vi "Write tSensorOnTreeElements_Core.vi"(8 "error in (no error)":errorcluster, 9 "System_settings IN":T1={"Units in the system"=[], "dBase names by units"=[], "TCP/IP processing units addresses"=[], "TCP/IP server address"="", "dBase User Name_Cli"="codis_cli", "dBase User Password_Cli"="codis_cli", "dBase User Name_Med"="codis_med_wrt", "dBase User Password_Med"="codis_med_wrt", "Sampling rate [Hz]"=0.0, "FTP Server User name, cRIO"="", "FTP Server Password, cRIO"="", "OnScreenKeyboardPopUp"=FALSE, "Number of points to collect"=0, "Main Window has title bar?"=FALSE, "Demo?"=FALSE, "dBase - Limit # of  elements to read"=0, "dBase Backup"={"dBase Backup Base Folder"="c:\\codis\\backup\\", "Remote dBase Backup Configured?"=TRUE}, "System Status"={"System Monitor Refresh Rate (ms)"=10000, "System Status Log  File"="c:\\codis\\system_info.txt", "Max number of elements to read\n"=26611200}, "Number of points to average for stationary state"=[60], "Number of points to collect for saving waveforms per channel"=[60], "Sources per Unit"=[], "TCP/IP_client_mediator_communication ports"=2058, "TCP/IP processing_units _mediator_communication ports"=2055}, 11 "1D array of Waveform Cluster IN":T4[](array[typedef]) {"Analysis Parameters"."SP2Pmax"."Filter Parameters"."low cutoff freq: fl" format="%0.4f"; "Analysis Parameters"."SP2Pmax"."Filter Parameters"."high cutoff freq: fh" format="%0.2f"; "Analysis Parameters"."LoadAngleDelta"."Multiplication Factor" format="%.1f"; "Analysis Parameters"."LoadAngleDelta"."What harmonic? (for example 24th (48 pole machine))" format="%.1f"; "Analysis Parameters"."Peak2Peak"."Filter Parameters"."low cutoff freq: fl" format="%0.4f"; "Analysis Parameters"."Peak2Peak"."Filter Parameters"."high cutoff freq: fh" format="%0.2f"; "Analysis Parameters"."RMS"."Filter Parameters"."order" format="%0.4f"; "Analysis Parameters"."RMS"."Filter Parameters"."low cutoff freq: fl" format="%0.2f"; "Analysis Parameters"."RMS"."Filter Parameters"."high cutoff freq: fh" format="%0.2f"; "Analysis Parameters"."EqPeak"."Filter Parameters"."low cutoff freq: fl" format="%0.4f"; "Analysis Parameters"."EqPeak"."Filter Parameters"."high cutoff freq: fh" format="%0.2f"; "Analysis Parameters"."Peak"."Filter Parameters"."low cutoff freq: fl" format="%0.4f"; "Analysis Parameters"."Peak"."Filter Parameters"."high cutoff freq: fh" format="%0.2f"; "Analysis Parameters"."snPh"."What harmonic?" format="%.1f"; "Analysis Parameters"."snA"."Multiplication Factor" format="%.1f"; "Analysis Parameters"."snA"."What harmonic?" format="%.1f"; "Analysis Parameters"."Smax"."Filter Parameters"."low cutoff freq: fl" format="%0.4f"; "Analysis Parameters"."Smax"."Filter Parameters"."high cutoff freq: fh" format="%0.2f"; "Analysis Parameters"."RPM"."Signal Threshold" format="%.1f"}) -> ()   [LabVIEW 2014]
uses:
  common/typedefs/Waveforms_Cluster_Core.ctl
  common/typedefs/Unit_Names_Core.ctl
  common/typedefs/Data_Sources_Core.ctl
  common/typedefs/Types_of_Signals_Core.ctl
  common/typedefs/Types_of_Analyses_Core.ctl
  common/typedefs/Analysis_Parameters_Cluster_Core.ctl
  <vilib>/Analysis/3filter.llb/Filter Passband Type.ctl
  common/typedefs/Integration_Types_Core.ctl
  common/typedefs/System_Settings_Cluster_Client_Mediator_Core.ctl
  <vilib>/addons/database/Connection.llb/DB Tools Open Connec (String).vi
  <vilib>/addons/database/NI_Database_API.lvlib
  <vilib>/Analysis/NI_AALBase.lvlib
panel:
  out "error out 2":errorcluster
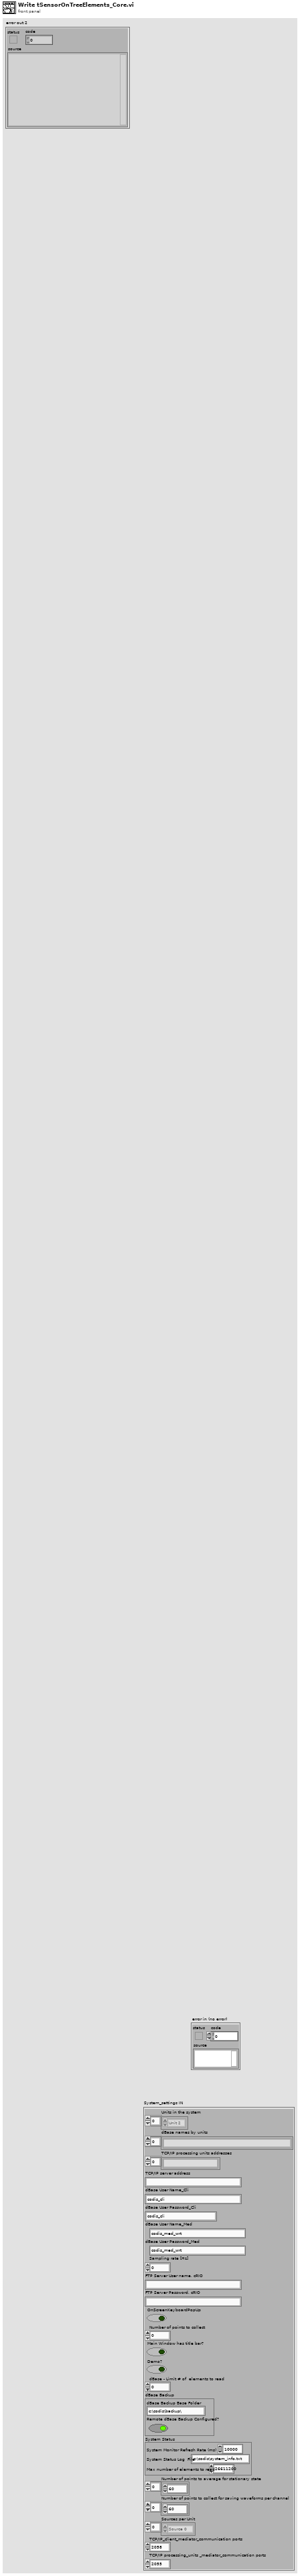
[diagram p1: front panel]
types:
  T1 = typedef "System_Settings_Cluster_Client_Mediator_Core.ctl" = cluster{"Units in the system":T2[], "dBase names by units":string[], "TCP/IP processing units addresses":string[], "TCP/IP server address":string, "dBase User Name_Cli":string, "dBase User Password_Cli":string, "dBase User Name_Med":string, "dBase User Password_Med":string, "Sampling rate [Hz]":dbl, "FTP Server User name, cRIO":string, "FTP Server Password, cRIO":string, "OnScreenKeyboardPopUp":bool, "Number of points to collect":u32, "Main Window has title bar?":bool, "Demo?":bool, "dBase - Limit # of  elements to read":u32, "dBase Backup":cluster{"dBase Backup Base Folder":string, "Remote dBase Backup Configured?":bool}, "System Status":cluster{"System Monitor Refresh Rate (ms)":u32, "System Status Log  File":string, "Max number of elements to read\n":i64}, "Number of points to average for stationary state":i32[], "Number of points to collect for saving waveforms per channel":i32[], "Sources per Unit":T3[], "TCP/IP_client_mediator_communication ports":u16, "TCP/IP processing_units _mediator_communication ports":u16}
  T2 = typedef "Unit_Names_Core.ctl" = enum16{"Not used", "Unit 1", "Unit 2", "Unit 3", "Unit 4", "Unit 5", "Unit 6", "Unit 7", "Unit 8", "Unit 9"}
  T3 = typedef "Data_Sources_Core.ctl" = enum16{"Not Used", "Source 0", "Source 1", "Source 2", "Source 3", "Source 4", "Source 5", "Source 6", "Source 7", "Source 8", "Source 9", "Source 10", "Source 11", "Source 12", "Source 13", "Source 14", "Source 15", "Source 16", "Source 17", "Source 18", "Source 19", "Source 20"}
  T4 = typedef "Waveforms_Cluster_Core.ctl" = cluster{"Configuration File loaded successfully? ":bool, "Is this new configuration?":bool, "Unit Name":T2, "Waveform Source":T3[], "Use CoDiS server Timestamp (on FALSE uses Processing Unit Timestamp)?":bool, "Sampling Rate [Hz]":u32[], "Timestamp (DBL)":dbl, "Mode of Operation - Normal":string, "Mode of Operation - Diagnostic":string, "Waveform Physical Channel":u16[], "Waveform Label":string[], "Waveform Name":string[], "Signal Type":cluster{"Signal Type":T5, "# of signal of particular type":u8}[], "Is this Main Trigger Signal?":bool[], "Slope":dbl[], "Intercept":dbl[], "Waveform Values":sgl[][], "Analyse?":bool[], "Save to database?":bool[], "Analyses to Perform":T6[][], "Perform this analysis on a CoDiS server?":bool[][], "General Parameters":cluster{"Number of Poles":u8, "Grid Frequency":sgl}, "Analysis Parameters":T7[][], "Save now to dBase?":bool, "Waveform Length for Saving [s]":u16, "Pretrigger Length when Saving Waveform [s]":u16, "Next Timestamp to autosave at (DBL)":dbl, "Description of Waveforms Events":string, "Event Type":string, "Save next RS event entirely? (on FALSE uses How many basic (acquisition) blocks of data (loops) to save?":bool, "Regime Name for which to save next RS event entirely":string, "Integration type":T9[], "Channel not OK?":bool[], "Channel Not OK?  Relay Number (-1 = none, 0, ..., MAX)":i16[], "Array of FPGA Filter Parameters":cluster{"Filter signal?":bool, "filter type":T8, "high cutoff freq: fh":dbl, "low cutoff freq: fl":dbl, "order":i32}[][], "Pre-Alarm Delay in Number of Loops ":u16, "Pre-Trip Delay in Number of Loops ":u16}
  T5 = typedef "Types_of_Signals_Core.ctl" = enum16{"Not Used", "Trigger (TRG???)", "Relative Vibrations (RV???)", "Absolute Vibrations (AV???)", "Air Gap (AG???)", "Magnetic Field (MX???)", "Voltage (VOL???)", "Current (CURR???)", "Process (PROC???)", "Cavitation (CAV???)", "Non Standard (NONST???)", "Axial Displacement (AXD???)", "Absolute Vibrations Stator Core (AVSC???)"}
  T6 = typedef "Types_of_Analyses_Core.ctl" = enum16{"Exit Analysis Loop", "Do Nothing", "RPM", "Smax", "SP2Pmax", "snA", "snPh", "Rest", "Peak", "EqPeak", "Peak2Peak", "RMS", "DC", "DC from Extrema", "Min Value", "Max Value", "Min Value by Pole", "Max Value by Pole", "Max Diff by Pole", "Max Diff Pole Number", "Min from Extrema", "Max from Extrema", "Active Power from DFT", "Active Power by Integration", "Reactive Power from DFT", "Reactive Power by Integration", "Apparent Power", "Ampl@Freq", "Phase Difference", "Load Angle Delta", "THD", "Signal Frequency", "Eta", "Non standard (CoDiS server - manual) 0", "Non standard (CoDiS server - manual) 1", "Non standard (CoDiS server - manual) 2", "Non standard (CoDiS server - manual) 3", "Non standard (CoDiS server - manual) 4", "Non standard (CoDiS server - manual) 5", "Non standard (CoDiS server - manual) 6", "Non standard (CoDiS server - manual) 7", "Non standard (CoDiS server - manual) 8", "Non standard (CoDiS server - manual) 9", "Non standard (CoDiS server - manual) 10", "Non standard (CoDiS server - manual) 11", "Non standard (CoDiS server - manual) 12", "Non standard (CoDiS server - manual) 13", "Non standard (CoDiS server - manual) 14", "Non standard (CoDiS server - manual) 15", "Non standard (CoDiS server - manual) 16", "Non standard (CoDiS server - manual) 17", "Non standard (CoDiS server - manual) 18", "Non standard (CoDiS server - manual) 19", "CosFi", "Total THD", "Crest Factor"}
  T7 = typedef "Analysis_Parameters_Cluster_Core.ctl" = cluster{"DC":cluster{"Analyze data from 1st trigger to last (if possible)? (FALSE=analyze everything)":bool}, "DCExtrema":cluster{"Calculate DC from all Pole Values":bool, "Poles to use in DC calculation (if Calculate DC from all Pole Values is FALSE)":u8[], "Condition Vector Label begin Part (MinPole or MaxPole)":string, "Addition to Condition Vector Label (example: 000)":string}, "RPM":cluster{"Signal Threshold":sgl, "Pulse Width (should be >= 2 depending on signal noise)":i32, "Trigger on rising edge? (FALSE=trigger on falling)":bool}, "Smax":cluster{"Combine with which Waveform Label? (for example: RV001)":string, "Calculate from time-averaged signal on one revolution?":bool, "Analyze data from 1st trigger to last (if possible)? (FALSE=analyze everything)":bool, "Filter Parameters":cluster{"Filter signal?":bool, "filter type":T8, "high cutoff freq: fh":dbl, "low cutoff freq: fl":dbl, "order":i32, "Process as ring-buffer signal?":bool}, "Gliding Parameters":cluster{"Glide signal?":bool, "Number of points for gliding":u16}, "Average all calculated values for Smax - if present (each revolution)? (FALSE=take absolute maximum)":bool, "Addition to Condition Vector Label (example: 000)":string}, "SP2Pmax":cluster{"Combine with which Waveform Label? (for example: RV001)":string, "Calculate from time-averaged signal on one revolution?":bool, "Analyze data from 1st trigger to last (if possible)? (FALSE=analyze everything)":bool, "Filter Parameters":cluster{"Filter signal?":bool, "filter type":T8, "high cutoff freq: fh":dbl, "low cutoff freq: fl":dbl, "order":i32, "Process as ring-buffer signal?":bool}, "Gliding Parameters":cluster{"Glide signal?":bool, "Number of points for gliding":u16}, "Average all calculated values for SP2Pmax - if present (each revolution)? (FALSE=take absolute maximum)":bool, "Addition to Condition Vector Label (example: 000)":string}, "snA":cluster{"What harmonic?":sgl, "Calculate Amplitude (TRUE) or RMS (FALSE)?":bool, "Multiplication Factor":sgl, "Calculate Amplitude for Air Gap type signals? (from MinPole Values)":bool}, "snPh":cluster{"What harmonic?":sgl}, "Peak":cluster{"Calculate from time-averaged signal (one-revolution)?":bool, "Analyze data from 1st trigger to last (if possible)? (FALSE=analyze everything)":bool, "Filter Parameters":cluster{"Filter signal?":bool, "filter type":T8, "high cutoff freq: fh":dbl, "low cutoff freq: fl":dbl, "order":i32, "Process as ring-buffer signal?":bool}, "Gliding Parameters":cluster{"Glide signal?":bool, "Number of points for gliding":u16}, "Average all calculated values for Peak - if present (each revolution)? (FALSE=take absolute maximum)":bool, "Addition to Condition Vector Label (example: 000)":string}, "Peak2Peak":cluster{"Calculate from time-averaged signal (one-revolution)?":bool, "Analyze data from 1st trigger to last (if possible)? (FALSE=analyze everything)":bool, "Gliding Parameters":cluster{"Glide signal?":bool, "Number of points for gliding":u16}, "Filter Parameters":cluster{"Filter signal?":bool, "filter type":T8, "high cutoff freq: fh":dbl, "low cutoff freq: fl":dbl, "order":i32, "Process as ring-buffer signal?":bool}, "Average all calculated values for Peak2Peak - if present (each revolution)? (FALSE=take absolute maximum)":bool, "Addition to Condition Vector Label (example: 000)":string}, "EqPeak":cluster{"Calculate from time-averaged signal (one-revolution)?":bool, "Analyze data from 1st trigger to last (if possible)? (FALSE=analyze everything)":bool, "Average all calculated values for EqPeak - if present (each revolution)? (FALSE=take absolute maximum)":bool, "Filter Parameters":cluster{"Filter signal?":bool, "filter type":T8, "high cutoff freq: fh":dbl, "low cutoff freq: fl":dbl, "order":i32, "Process as ring-buffer signal?":bool}, "Which Condition Vector Label addition to use for RMS (example: 001)":string, "Addition to Condition Vector Label (example: 000)":string}, "RMS":cluster{"Calculate from time-averaged signal (one-revolution)?":bool, "Analyze data from 1st trigger to last (if possible)? (FALSE=analyze everything)":bool, "Subtract DC before RMS calculation?":bool, "Filter Parameters":cluster{"Filter signal?":bool, "filter type":T8, "high cutoff freq: fh":dbl, "low cutoff freq: fl":dbl, "order":i32, "Process as ring-buffer signal?":bool}, "Gliding Parameters":cluster{"Glide signal?":bool, "Number of points for gliding":u16}, "Average all calculated values for RMS - if present (each revolution)? (FALSE=take absolute maximum)":bool, "Addition to Condition Vector Label (example: 000)":string}, "Rest":cluster{"Calculate from all calculated harmonics?":bool, "Condition Vector Label to use for substraction (if Calculate from all calculated harmonics?=FALSE)":string[], "Calculate by subtracting from EqPeak Value? (FALSE=calculate by subtracting from RMS Value)":bool, "Which Condition Vector Label addition to use for EqPeak (example: 001)":string, "Addition to Condition Vector Label (example: 000)":string}, "MinByPole":cluster{"First Pole Number after Trigger (indexes correspond to Normal regime settings)":u8[], "Are Pole Numbers in ascending order in time?  (indexes correspond to Normal regime settings)":bool[], "Average all calculated values for that Pole? (FALSE=take absolute minimum)":bool, "Coerce Upper Limit":sgl, "Compensate 1st harmonic in waveform?":bool}, "MinExtrema":cluster{"Calculate Min Extrema from all Pole Values":bool, "Poles to use in Min Extrema calculation (if Calculate Min Extrema from all Pole Values is FALSE)":u8[], "Condition Vector Label begin Part (MinPole or MaxPole)":string}, "MaxByPole":cluster{"First Pole Number after Trigger (indexes correspond to Normal regime settings)":u8[], "Are Pole Numbers in ascending order in time? (indexes correspond to Normal regime settings)":bool[], "Average all calculated values for that Pole? (FALSE=take absolute maximum)":bool, "Calculate with abs(Signal)?":bool, "Subtract DC before calculation?":bool, "Coerce Lower Limit":sgl}, "MaxExtrema":cluster{"Calculate Max Extrema from all Pole Values":bool, "Poles to use in Max Extrema calculation (if Calculate Max Extrema from all Pole Values is FALSE)":u8[], "Condition Vector Label begin Part (MinPole or MaxPole)":string}, "MaxDiffByPole":cluster{"First Pole Number after Trigger (indexes correspond to Normal regime settings)":u8[], "Are Pole Numbers in ascending order in time? (indexes correspond to Normal regime settings)":bool[], "Condition Vector Label begin Part (MinPole or MaxPole)":string}, "Min":cluster{"Analyze data from 1st trigger to last (if possible)? (FALSE=analyze everything)":bool, "Calculate from time-averaged signal on one revolution?":bool, "Gliding Parameters":cluster{"Glide signal?":bool, "Number of points for gliding":u16}, "Average all calculated values for Min - if present (each revolution)? (FALSE=take absolute maximum)":bool}, "Max":cluster{"Analyze data from 1st trigger to last (if possible)? (FALSE=analyze everything)":bool, "Calculate from time-averaged signal on one revolution?":bool, "Gliding Parameters":cluster{"Glide signal?":bool, "Number of points for gliding":u16}, "Average all calculated values for Max - if present (each revolution)? (FALSE=take absolute maximum)":bool}, "ActivePower":cluster{"Calculate from Phase Voltages and Currents?":bool, "Phase Voltage Condition Vector Label (R, S, T) (for example: VOL000.s24.00A, VOL001.s24.00A, VOL002.s24.00A)":string[], "Phase Current Condition Vector Label (R, S, T) (for example: CURR000.s24.00A, CURR001.s24.00A, CURR002.s24.00A)":string[]}, "ReactivePower":cluster{"Calculate from Phase Voltages and Currents?":bool, "Phase Voltage Condition Vector Label (R, S, T) (for example: VOL000.s24.00A, VOL001.s24.00A, VOL002.s24.00A)":string[], "Phase Current Condition Vector Label (R, S, T) (for example: CURR000.s24.00A, CURR001.s24.00A, CURR002.s24.00A)":string[]}, "LoadAngleDelta":cluster{"What harmonic? (for example 24th (48 pole machine))":sgl, "Delta0":sgl, "Which Voltage Waveform Label? (for example: VOL000)":string, "Combine (multiply) with which Air Gap Waveform Label? (for example: AG000)":string, "Multiplication Factor":sgl}, "ActivePowerByIntegration":cluster{"Phase Voltage Waveform Labels (R,S,T)":string[], "Phase Current Waveform Labels (R,S,T)":string[], "Analyze data from 1st trigger to last (if possible)? (FALSE=analyze everything)":bool}, "RectivePowerByIntegration":cluster{"Phase Voltage Waveform Vector Labels (R,S,T)":string[], "Phase Current Waveform Labels (R,S,T)":string[], "System Electric Frequency [Hz]":sgl, "Analyze data from 1st trigger to last (if possible)? (FALSE=analyze everything)":bool}, "Ampl@Freq":cluster{"Frequency [Hz]":sgl, "Calculate Amplitude? (FALSE=calculate RMS)":bool}, "PhaseDifference":cluster{"Combine with which Waveform Label?":string}, "CosFi":cluster{"Voltage Waveform Labels (R,S,T)":string[], "Current Waveform Labels (R,S,T)":string[]}, "Total THD":cluster{"THD Condition Vector Label (R, S, T) (for example: VOL000.THD, VOL001.THD, VOL002.THD)":string[]}, "Crest Factor":cluster{"Addition to Condition Vector Label (example: 000)":string, "Which Condition Vector Label addition to use for Peak (example: 001)":string, "Which Condition Vector Label addition to use for RMS (example: 001)":string}}
  T8 = typedef "NI_AALBase.lvlib/Filter Passband Type.ctl" = enum32{"Lowpass", "Highpass", "Bandpass", "Bandstop"}
  T9 = typedef "Integration_Types_Core.ctl" = enum16{"Do not integrate", "Integrate once", "Integrate twice"}
  T10 = typedef "NI_Database_API.lvlib/Conn ObjectReference.ctl" = refnum<k1>
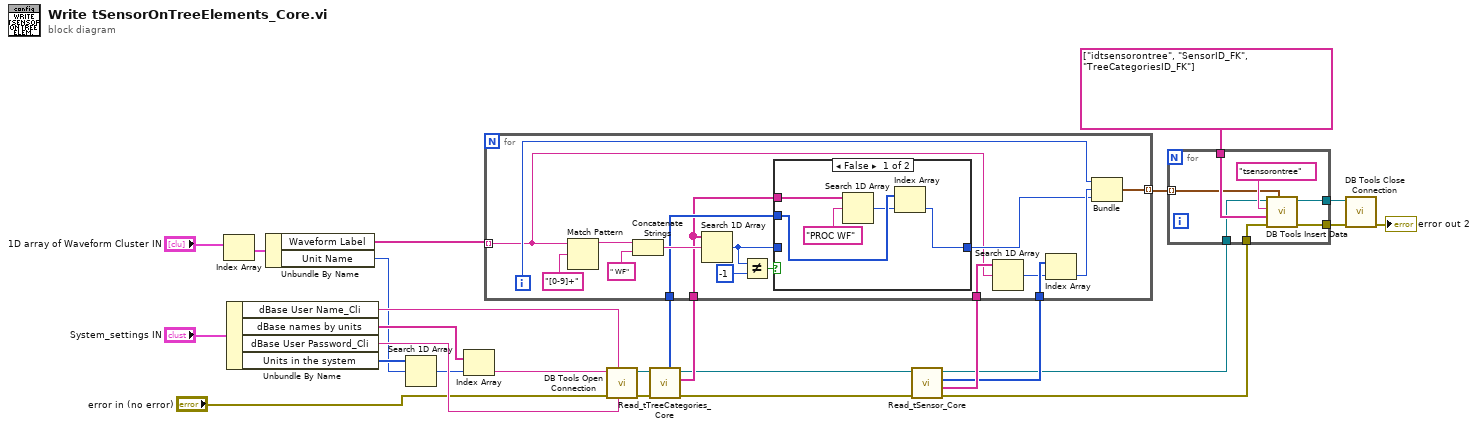
[diagram p0: block diagram]
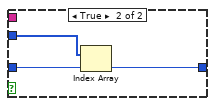
[diagram p2: hidden frame]
diagram:
  n1 = Index Array(array="1D array of Waveform Cluster IN") -> (element=w27:T4)  [unwired: 1 in]
  n2 = Unbundle By Name("System_settings IN") -> ("dBase User Name_Cli"=w22:string, "dBase names by units"=w23:string[], "dBase User Password_Cli"=w21:string, "Units in the system"=w20:T2[])
  n3 = Unbundle By Name(w27) -> ("Waveform Label"=w26:string[], "Unit Name"=w8:T2)
  n4 = Search 1D Array(1D array=w20, element=w8) -> (index of element=w19:i32)  [unwired: 1 in]
  n5 = Index Array(array=w23, index=w19) -> (element=w24:string)
  n6 = call-poly <vilib>:"DB Tools Open Connection.vi"("password"=w21, "userID"=w22, "error in (no error)"="error in (no error)", "connection information"=w24) -> ("error out"=w17:errorcluster, "connection reference"=w18:T10)  [unwired: 4 in]
  n7 = call "Read_tTreeCategories_Core.vi"("error in (no error)"=w17, "connection reference IN"=w18) -> ("error out"=w13:errorcluster, "TrreCategoryLabel"=w16:string[], "connection reference out"=w14:T10, "idtTreeCategories OUT"=w15:u32[])  [unwired: 4 in, 2 out]
  n8 = call "Read_tSensor_Core.vi"("error in (no error)"=w13, "connection reference IN"=w14) -> ("error out"=w6:errorcluster, "SensorLabel OUT"=w12:string[], "idtSensor OUT"=w11:u8[], "connection reference out"=w7:T10)  [unwired: 5 in, 1 out]
  n9 = for {
    tunnel: w26 -> [w33] mode=indexing
    tunnel: w16 -> [w28]
    tunnel: w15 -> [w42]
    tunnel: w12 -> [w41]
    tunnel: w11 -> [w39]
    tunnel: [w35] -> w10 mode=indexing
    i -> [w40]
    n10 = Match Pattern(string=w33, regular expression="[0-9]+") -> (before substring=w32:string)  [unwired: 1 in, 3 out]
    n11 = Concatenate Strings(w32, " WF" ("string")) -> (w43:string)
    n12 = Search 1D Array(1D array=w28, element=w43) -> (index of element=w31:i32)  [unwired: 1 in]
    n13 = Not Equal?(x=w31, y=-1) -> (x != y?=w29:bool)
    n14 = case shown="False" w29 {
      tunnel: w42 -> [w47 w52]
      tunnel: [w45 w51] -> w36
      tunnel: w31 -> [_ w50]
      tunnel: w28 -> [w49 _]
      frame False {
        n15 = Search 1D Array(1D array=w49, element="PROC WF" ("string")) -> (index of element=w46:i32)  [unwired: 1 in]
        n16 = Index Array(array=w47, index=w46) -> (element=w45:u32)
      }
      frame True {
        n17 = Index Array(array=w52, index=w50) -> (element=w51:u32)
      }
    }
    n18 = Search 1D Array(1D array=w41, element=w33) -> (index of element=w38:i32)  [unwired: 1 in]
    n19 = Index Array(array=w39, index=w38) -> (element=w37:u8)
    n20 = Bundle(w40, "data"=w37, "data"=w36) -> (w35:cluster{i32, "data":u8, "data":u32})  [unwired: 1 in]
  }
  n21 = for {
    tunnel: string[] ["idtsensorontree", "SensorID_FK", "TreeCategoriesID_FK"] ("columns") -> [w58]
    tunnel: w7 -> [w57]
    tunnel: w6 -> [w56]
    tunnel: [w55] -> w4
    tunnel: w10 -> [w54] mode=indexing
    tunnel: [w53] -> w5
    n22 = call <vilib>:"DB Tools Insert Data.vi"("data"=w54, "error in (no error)"=w56, "columns"=w58, "table"="tsensorontree", "connection reference"=w57) -> ("error out"=w55:errorcluster, "connection reference out"=w53:T10)  [unwired: 5 in]
  }
  n23 = call <vilib>:"DB Tools Close Connection.vi"("error in (no error)"=w4, "connection reference"=w5) -> ("error out"=→"error out 2":errorcluster)  [unwired: 5 in]
